vi "超音波資料擷取系統_平均值_用在波破碎.vi"() -> ()   [LabVIEW 2014]
uses:
  <vilib>/addons/database/Auxilliary.llb/DB Tools Column Info.ctl
  <vilib>/addons/database/Auxilliary.llb/DB Tools DataTypes.ctl
  <vilib>/addons/database/Connection.llb/DB Tools Open Connec (Path).vi
  <vilib>/Utility/file.llb/Write To Spreadsheet File (DBL).vi
  <vilib>/addons/database/Connection.llb/Conn Execute.vi
  <vilib>/addons/database/Recordset.llb/Rec Destroy - Connection.vi
  <vilib>/addons/database/NI_Database_API.lvlib
panel:
  out "data_average":dbl[][](array[numeric])
  out "a":dbl[][](array[numeric])
  out "Sum":dbl[][](array[numeric])
  out "data":dbl[][](array[numeric])
  in  "lowest value":dbl=4.0
  out "new file path (Not A Path if cancelled)":path
  out "new file path (Not A Path if cancelled) 2":path
  in  "average number":i16=200
  out "new file path (Not A Path if cancelled) 3":path
  out "Raw data 2":dbl[][](graph)
  out "transposed array":dbl[][](array[numeric])
  out "size(s)":i32[](array[numeric])
  out "table name":string
  in  "you name it":string="N波校正"
  out "Numeric":i32
  out "time/data array":string[][](array[string])
  out "data array size":i32[](array[numeric])
  out "assistant error":errorcluster
  out "Raw data":dynamicdata(graph)
  in  "stop":bool
  out "close error":errorcluster
  out "free error":errorcluster
  out "execute error":errorcluster
  out "create table error":errorcluster
  out "insert query array":string[](array[string])
  out "insert table( )":string
  out "array after delete":string[][](array[string])
  out "table column after delete":T1[](array[typedef])
  in  "connection path":path=path "C:/Program Files (x86)/National Instruments/LabVIEW 2014/Database/odbcmysql.udl"
  out "column of delete":dbl
  out "data array":string[][](array[string])
  in  "channel 3":bool=TRUE
  in  "channel 2":bool
  in  "channel 1":bool=TRUE
  in  "channel 0":bool=TRUE
  in  "rate":i32=5000
  in  "number of sample":i32=2500
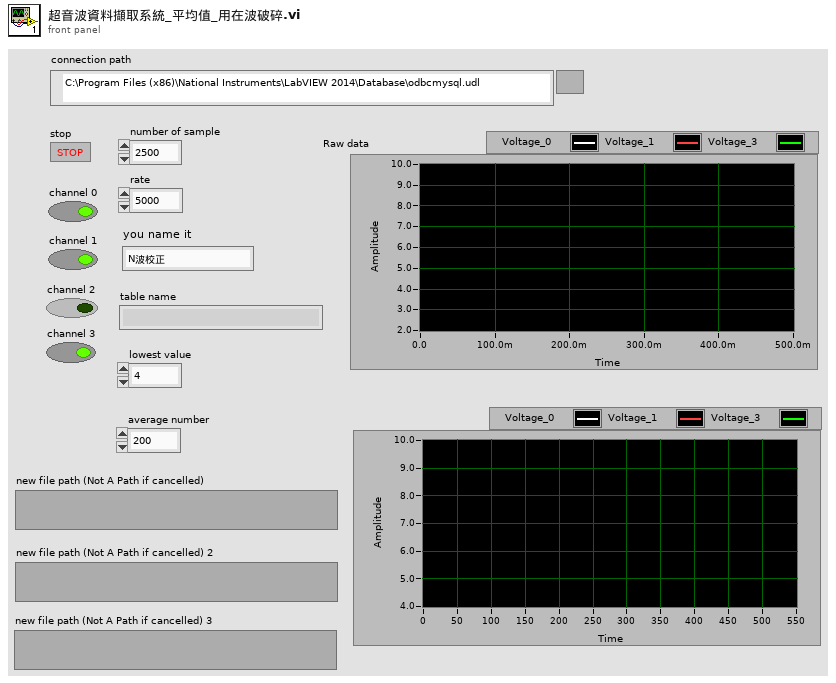
[diagram p1: front panel]
types:
  T1 = typedef "NI_Database_API.lvlib/DB Tools Column Info.ctl" = cluster{"column name":string, "data type":T2, "size":i32, "allow null?":bool}
  T2 = typedef "NI_Database_API.lvlib/DB Tools DataTypes.ctl" = enum16{"String", "Long (I32)", "Single (SGL)", "Double (DBL)", "Date/Time", "Binary"}
  T3 = cluster{"channel 0":bool, "channel 1":bool, "channel 2":bool, "channel 3":bool}
  T4 = typedef "NI_Database_API.lvlib/Conn ObjectReference.ctl" = refnum<k1>
  T5 = typedef "NI_Database_API.lvlib/Rec ObjectReference.ctl" = refnum<k1>
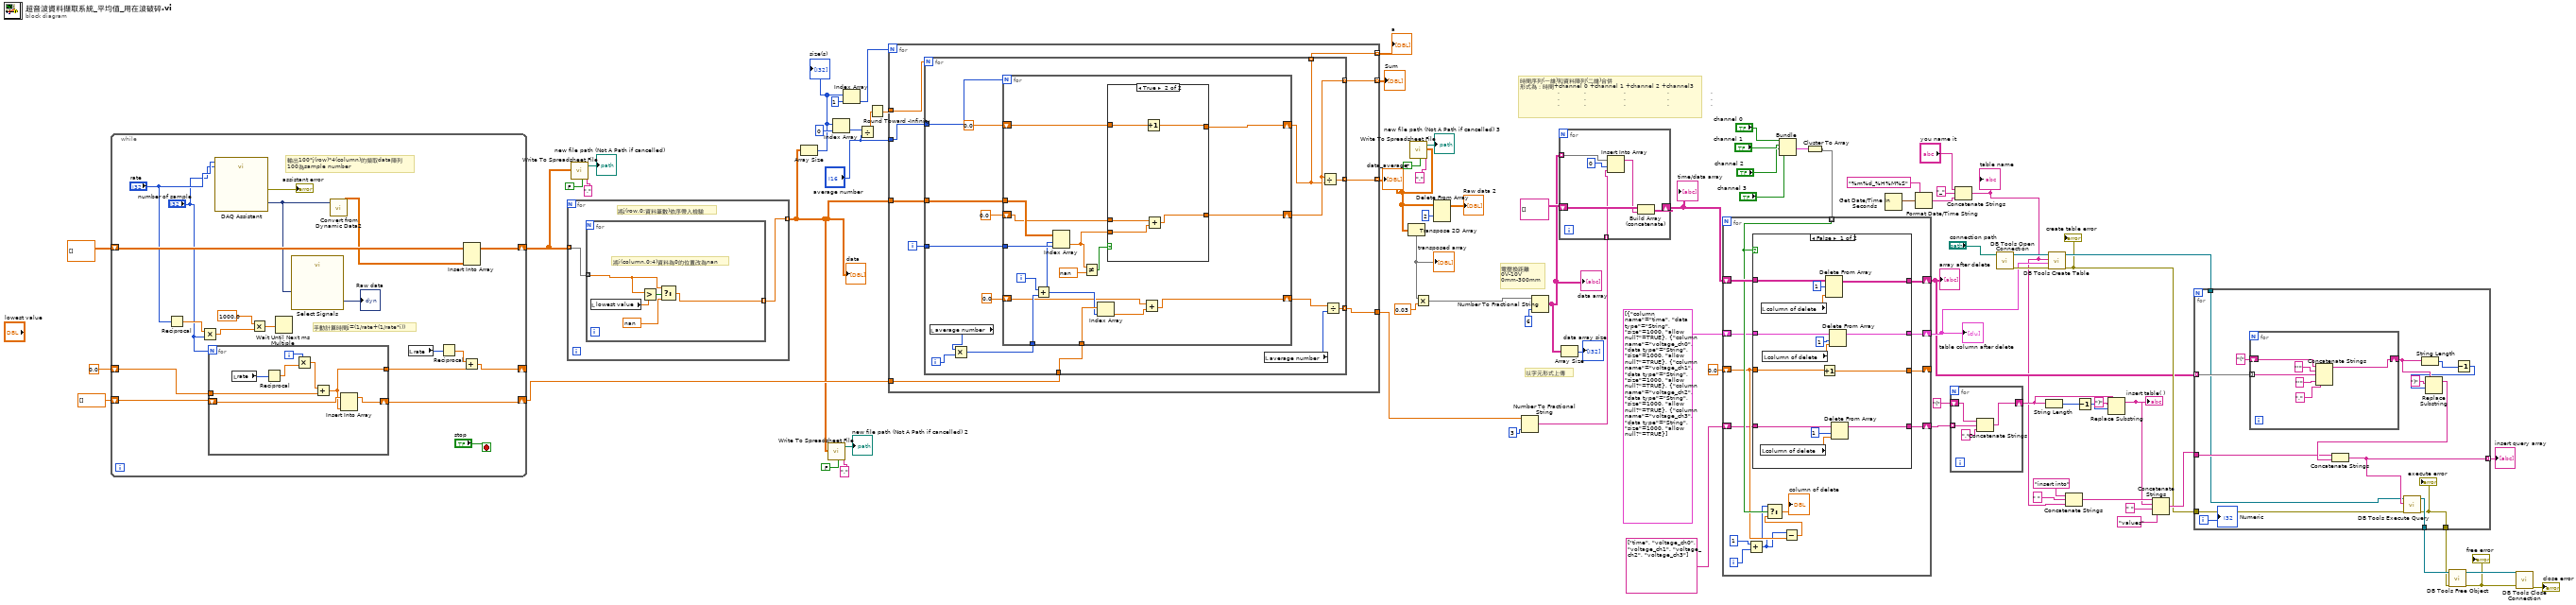
[diagram p0: block diagram]
diagram:
  # "以字元形式上傳"
  # "電壓換距離\n0V-10V\n0mm-300mm"
  # "時間序列(一維)和資料陣列(二維)合併 \n形式為：時間+channel 0 +channel 1 +channel 2 +channel3\n                    .             .                    .                      .                      .\n                    .             .                    .                      .                      .\n                    .             .                    .                      .                      ."
  n1 = while {
    shift-right: [w87] -> w10
    shift-left: dbl[][] [] -> [w98]
    shift-right: [w93] -> w23
    shift-left: dbl[] [] ("array") -> [w94]
    shift-right: [w88] -> _
    shift-left: 0.0 -> [w92]
    stop <- "stop" stop-if-true
    # "手動計算時間j=(1/rate+(1/rate*i))"
    # "輸出100*j(row)*4(column)的擷取data陣列\n100為sample number"
    n2 = Reciprocal(x="rate") -> (1/x=w96:dbl)
    n3 = Multiply(x=w96, y="number of sample") -> (x*y=w99:dbl)
    n4 = for {
      N: "number of sample" -> [_]
      shift-right: [w104] -> w93
      shift-left: w94 -> [w103]
      tunnel: w92 -> [w102]
      tunnel: [w101] -> w91
      i -> [w107]
      n5 = local read "rate"() -> (w108:i32)
      n6 = Reciprocal(x=w108) -> (1/x=w106:dbl)
      n7 = Multiply(x=w107, y=w106) -> (x*y=w105:dbl)
      n8 = Add(x=w105, y=w102) -> (x+y=w101:dbl)
      n9 = Insert Into Array(array=w103, new element=w101) -> (w104:dbl[])  [unwired: 1 in]
    }
    n10 = call "DAQ Assistant"("rate"="rate", "number of samples"="number of sample") -> ("data"=w82:dynamicdata, "error out"=→"assistant error":errorcluster)  [unwired: 14 in, 2 out]
    n11 = Multiply(x=1000.0 ("y"), y=w99) -> (x*y=w95:dbl)
    n12 = Wait Until Next ms Multiple(millisecond multiple=w95) -> ()  [unwired: 1 out]
    n13 = call "Select Signals"("Signals"=w82) -> ("Signal Out"=→"Raw data":dynamicdata)  [unwired: 9 in, 1 out]
    n14 = call "Convert from Dynamic Data2"("Dynamic Data Type"=w82) -> ("Array"=w86:dbl[][])  [unwired: 3 in]
    n15 = local read "rate"() -> (w89:i32)
    n16 = Reciprocal(x=w89) -> (1/x=w90:dbl)
    n17 = Insert Into Array(array=w98, new element=w86) -> (w87:dbl[][])  [unwired: 2 in]
    n18 = Add(x=w90, y=w91) -> (x+y=w88:dbl)
  }
  n19 = for {
    tunnel: w10 -> [w110] mode=indexing
    tunnel: [w109] -> w1 mode=indexing
    # "將j(row,0:資料筆數)依序帶入檢驗"
    n20 = for {
      tunnel: w110 -> [w113] mode=indexing
      tunnel: [w112] -> w109 mode=indexing
      # "將i(column,0:4)資料為0的位置改為nan"
      n21 = local read "lowest value"() -> (w111:dbl)
      n22 = Greater?(x=w113, y=w111) -> (0:w114:bool)
      n23 = Select(t=w113, s=w114, f=nan) -> (s? t:f=w112:dbl)
    }
  }
  "data" <- w1
  n24 = call-poly <vilib>:"Write To Spreadsheet File.vi"("delimiter (\\t)"="," ("delimiter (\\t)"), "transpose? (no:F)"=FALSE, "2D data"=w10) -> ("new file path (Not A Path if cancelled)"=→"new file path (Not A Path if cancelled)":path)  [unwired: 5 in]
  n25 = Array Size(array=w1) -> (size(s)=w25:i32[])
  "size(s)" <- w25
  n26 = call-poly <vilib>:"Write To Spreadsheet File.vi"("delimiter (\\t)"="," ("delimiter (\\t)"), "transpose? (no:F)"=FALSE, "2D data"=w1) -> ("new file path (Not A Path if cancelled)"=→"new file path (Not A Path if cancelled) 2":path)  [unwired: 5 in]
  n27 = Index Array(array=w25, index=0) -> (element=w27:i32)
  n28 = Index Array(array=w25, index=1) -> (element=w24:i32)
  n29 = Divide(x=w27, y="average number") -> (x/y=w5:dbl)
  n30 = Round Toward -Infinity(1:w5) -> (0:w4:dbl)
  n31 = for {
    N: w24 -> [_]
    tunnel: w1 -> [w124]
    tunnel: "average number" -> [w123]
    tunnel: w4 -> [w116]
    tunnel: [w121] -> w8 mode=indexing
    tunnel: w23 -> [w120]
    tunnel: [w119] -> w22
    tunnel: [w118] -> w3 mode=indexing
    tunnel: [w117] -> w2 mode=indexing
    i -> [w122]
    n32 = for {
      N: w116 -> [_]
      tunnel: w124 -> [w140]
      tunnel: w123 -> [w125]
      tunnel: w122 -> [w137]
      tunnel: [w134] -> w121 mode=indexing
      tunnel: w120 -> [w133]
      tunnel: [w130] -> w119 mode=indexing
      tunnel: [w127] -> w118 mode=indexing
      tunnel: [w126] -> w117 mode=indexing
      i -> [w139]
      n33 = local read "average number"() -> (w129:i16)
      n34 = Multiply(x=w129, y=w139) -> (x*y=w138:i32)
      n35 = for {
        N: w125 -> [_]
        tunnel: w140 -> [w149]
        tunnel: w138 -> [w154]
        tunnel: w137 -> [w153]
        shift-right: [w150] -> w126
        shift-left: 0.0 -> [w151]
        shift-right: [w142] -> w127
        shift-left: 0.0 -> [w143]
        shift-right: [w148] -> w131
        shift-left: 0.0 -> [w144]
        tunnel: w133 -> [w147]
        i -> [w155]
        n36 = Add(x=w155, y=w154) -> (x+y=w146:i32)
        n37 = Index Array(array=w149, index (row)=w146, index (col)=w153) -> (element=w141:dbl)
        n38 = Not Equal?(x=w141, y=nan) -> (x != y?=w152:bool)
        n39 = Index Array(array=w147, index=w146) -> (element=w145:dbl)
        n40 = case shown="True" w152 {
          tunnel: w151 -> [w158 w163]
          tunnel: [w158 w162] -> w150
          tunnel: w143 -> [w157 w161]
          tunnel: [w157 w160] -> w142
          tunnel: w141 -> [_ w159]
          frame False {
          }
          frame True {
            n41 = Increment(x=w163) -> (x+1=w162:dbl)
            n42 = Add(x=w161, y=w159) -> (x+y=w160:dbl)
          }
        }
        n43 = Add(x=w144, y=w145) -> (x+y=w148:dbl)
      }
      n44 = local read "average number"() -> (w128:i16)
      n45 = Divide(x=w127, y=w126) -> (x/y=w134:dbl)
      n46 = Divide(x=w131, y=w128) -> (x/y=w130:dbl)
    }
  }
  "Sum" <- w3
  "a" <- w2
  "data_average" <- w8
  n47 = Transpose 2D Array(2D array=w8) -> (transposed array=w9:dbl[][])
  "transposed array" <- w9
  n48 = call-poly <vilib>:"Write To Spreadsheet File.vi"("delimiter (\\t)"="," ("delimiter (\\t)"), "transpose? (no:F)"=TRUE, "2D data"=w8) -> ("new file path (Not A Path if cancelled)"=→"new file path (Not A Path if cancelled) 3":path)  [unwired: 5 in]
  n49 = Multiply(x=w9, y=0.03) -> (x*y=w18:dbl[][])
  n50 = Delete From Array(array=w8, index (row)=2) -> (array with subset deleted=→"Raw data 2":dbl[][])  [unwired: 2 in, 1 out]
  n51 = Number To Fractional String(number=w22, precision (6)=i16 3) -> (F-format string=w37:string[])  [unwired: 2 in]
  n52 = Number To Fractional String(number=w18, precision (6)=i16 6) -> (F-format string=w48:string[][])  [unwired: 2 in]
  "data array" <- w48
  n53 = for {
    shift-right: [w165] -> w47
    shift-left: string[][] [] -> [w167]
    tunnel: w48 -> [w168] mode=indexing
    tunnel: w37 -> [w164] mode=indexing
    n54 = Insert Into Array(array=w168, index=0, new element=w164) -> (w166:string[])
    n55 = Build Array (concatenate)(w167, w166) -> (w165:string[][])
  }
  "time/data array" <- w47
  n56 = Array Size(array=w48) -> (size(s)=→"data array size":i32[])
  n57 = Bundle("channel 0"="channel 0", "channel 1"="channel 1", "channel 2"="channel 2", "channel 3"="channel 3") -> (w74:T3)  [unwired: 1 in]
  n58 = Cluster To Array(cluster=w74) -> (array=w73:bool[])
  n59 = for {
    tunnel: w73 -> [w178] mode=indexing
    shift-right: [w182] -> w40
    shift-left: w47 -> [w183]
    shift-right: [w179] -> _
    shift-left: 0.0 -> [w177]
    shift-right: [w172] -> w50
    shift-left: T1[] [{"column name"="time", "data type"=enum."String", "size"=1000, "allow null?"=TRUE}, {"column name"="voltage_ch0", "data type"=enum."String", "size"=1000, "allow null?"=TRUE}, {"column name"="voltage_ch1", "data type"=enum."String", "size"=1000, "allow null?"=TRUE}, {"column name"="voltage_ch2", "data type"=enum."String", "size"=1000, "allow null?"=TRUE}, {"column name"="voltage_ch3", "data type"=enum."String", "size"=1000, "allow null?"=TRUE}] ("column information") -> [w173]
    shift-right: [w170] -> w68
    shift-left: string[] ["time", "voltage_ch0", "voltage_ch1", "voltage_ch2", "voltage_ch3"] -> [w171]
    i -> [w181]
    n60 = Add(x=1, y=w181) -> (x+y=w175:i32)
    n61 = case shown="False" w178 {
      tunnel: w183 -> [w197 w201]
      tunnel: [w196 w201] -> w182
      tunnel: w177 -> [w194 w199]
      tunnel: [w193 w199] -> w179
      tunnel: w173 -> [w191 w200]
      tunnel: [w190 w200] -> w172
      tunnel: w171 -> [w187 w198]
      tunnel: [w186 w198] -> w170
      frame False {
        n62 = local read "column of delete"() -> (w185:dbl)
        n63 = local read "column of delete"() -> (w192:dbl)
        n64 = local read "column of delete"() -> (w189:dbl)
        n65 = Increment(x=w194) -> (x+1=w193:dbl)
        n66 = Delete From Array(array=w197, length=1, index (col)=w192) -> (array with subset deleted=w196:string[][])  [unwired: 1 in, 1 out]
        n67 = Delete From Array(array=w191, length=1, index=w189) -> (array with subset deleted=w190:T1[])  [unwired: 1 out]
        n68 = Delete From Array(array=w187, length=1, index=w185) -> (array with subset deleted=w186:string[])  [unwired: 1 out]
      }
      frame True {
      }
    }
    n69 = Subtract(x=w175, y=w177) -> (x-y=w176:dbl)
    n70 = Select(t=w175, s=w178, f=w176) -> (s? t:f=→"column of delete":dbl)
  }
  "table column after delete" <- w50
  "array after delete" <- w40
  n71 = Get Date/Time In Seconds() -> (seconds since 1Jan1904=w32:timestamp)
  n72 = Format Date/Time String(time format string (%c)="%m%d_%H%M%S", seconds (now)=w32) -> (date/time string=w29:string)  [unwired: 1 in]
  n73 = for {
    tunnel: w68 -> [w204] mode=indexing
    shift-right: [w205] -> w62
    shift-left: "(" -> [w203]
    n74 = Concatenate Strings(w203, w204, "," ("string")) -> (w205:string)
  }
  n75 = Concatenate Strings("you name it", "_" ("string"), w29) -> (w33:string)
  "table name" <- w33
  n76 = call-poly <vilib>:"DB Tools Open Connection.vi"("connection information"="connection path") -> ("error out"=w56:errorcluster, "connection reference"=w70:T4)  [unwired: 7 in]
  n77 = String Length(string=w62) -> (length=w64:i32)
  n78 = call <vilib>:"DB Tools Create Table.vi"("error in (no error)"=w56, "column information"=w50, "table"=w33, "connection reference"=w70) -> ("error out"=w43:errorcluster, "connection reference out"=w44:T4)  [unwired: 4 in]
  "create table error" <- w43
  n79 = Concatenate Strings("insert into" ("string"), " " ("string"), w33) -> (w58:string)
  n80 = Decrement(x=w64) -> (x-1=w63:i32)
  n81 = Replace Substring(3:w63, 4:")" ("substring (\"\")"), 5:w62) -> (1:w49:string)  [unwired: 1 in, 1 out]
  "insert table( )" <- w49
  n82 = Concatenate Strings(w58, w49, " " ("string"), "values" ("string")) -> (w57:string)
  n83 = for {
    tunnel: w40 -> [w219] mode=indexing
    tunnel: w57 -> [w213]
    tunnel: [w211] -> w55 mode=indexing
    tunnel: [w210] -> w46
    tunnel: w44 -> [w209]
    tunnel: w43 -> [w208]
    tunnel: [w207] -> w42
    i -> [w206]
    n84 = for {
      shift-right: [w223] -> w218
      shift-left: "(" -> [w224]
      tunnel: w219 -> [w225] mode=indexing
      n85 = Concatenate Strings(w224, "'" ("string"), w225, "'" ("string"), "," ("string")) -> (w223:string)
    }
    n86 = String Length(string=w218) -> (length=w217:i32)
    n87 = Decrement(x=w217) -> (x-1=w216:i32)
    n88 = Replace Substring(3:w216, 4:")" ("substring (\"\")"), 5:w218) -> (1:w214:string)  [unwired: 1 in, 1 out]
    n89 = Concatenate Strings(w213, w214) -> (w211:string)
    n90 = call-poly <vilib>:"DB Tools Execute Query.vi"("error in (no error)"=w208, "SQL query"=w211, "connection reference"=w209) -> ("error out"=w207:errorcluster, "recordset reference"=w210:T5)  [unwired: 5 in]
    "execute error" <- w207
    "Numeric" <- w206
  }
  "insert query array" <- w55
  n91 = call-poly <vilib>:"DB Tools Free Object.vi"("error in (no error)"=w42, "recordset reference"=w46) -> ("error out"=w41:errorcluster, "connection reference"=w45:T4)  [unwired: 8 in]
  "free error" <- w41
  n92 = call <vilib>:"DB Tools Close Connection.vi"("error in (no error)"=w41, "connection reference"=w45) -> ("error out"=→"close error":errorcluster)  [unwired: 5 in]
